vi "Dashboard Main.vi"() -> ()   [LabVIEW 2013]
uses:
  <vilib>/event_ctls.llb/eventvkey.ctl
  <vilib>/Rock Robotics/WPI/Dashboard/WPI_DashboardLogging Global.vi
  <vilib>/Utility/config.llb/Write Key (String).vi
  <vilib>/Utility/config.llb/Write Key (I32).vi
  <vilib>/Utility/config.llb/NI_LVConfig.lvlib
panel:
  out "Image Message":string="Timeout in Camera Communications"
  in  "Rec Mode":enum32{"Stop", "Record", "Playback"}(radio)
  in  "Dashboard Tab":T1(tab)
  out "right Encoder":dbl
  out "left Encoder":dbl
  out "Mode":string
  out "Timer":dbl
  in  "Camera Settings":T2={"Frame Rate"=30, "Compression"=30, "Size"=1} {"Frame Rate" scale=1.0..30.0; "Size" items=["640x480", "320x240", "160x120"]}
  out "MotorSliders R":cluster{"MotorSlide1":dbl, "MotorSlide2":dbl} {"MotorSlide2" scale=-1.0..1.0 scale format="%#_2e"; "MotorSlide1" scale=-1.0..1.0 scale format="%#_2e"}
  out "MotorChart R":cluster{"Numeric":dbl, "Numeric":dbl}(graph)
  out "MotorSliders L":T3 {"MotorSlide4 2" scale=0.0..14.0 scale format="%#_2e"; "MotorSlide2" scale=-1.0..1.0 scale format="%#_2e"; "MotorSlide1" scale=-1.0..1.0 scale format="%#_2e"}
  out "MotorChart L":T4(graph)
  out "JS1 Z":dbl(slide) scale=-1.0..1.0 scale format="%#_2e"
  out "Joystick 1":cluster{"X":dbl, "Y":dbl}[](graph)
  out "JS Buttons 1":T5
  out "JS2 Z":dbl(slide) scale=-1.0..1.0 scale format="%#_2e"
  out "Joystick 2":cluster{"X":dbl, "Y":dbl}[](graph)
  out "JS Buttons 2":T5
  out "Mode":T6(ring)=enum."Auto Disabled"
  out "Camera IP":string
  in  "DB Camera Config":bool
  out "fps":dbl format="%#.1g"
  out "Mbps":dbl format="%#.1g"
  out "Mbps 2":bool
  out "LED 1":bool
  out "Polt 2 Ind":dbl
  out "Plot 1 Ind":dbl
  out "Plot 0 Ind":dbl
  out "Waveform Chart":T7(graph)
  in  "Checkbox 2":bool
  in  "Checkbox 1":bool
  in  "Test Slider":dbl(slide) scale=0.0..100.0 scale format="%#_3g"
  in  "On/Off":bool caption="Solenoid"
  in  "Test Name":u16(ring) items=["Select the test to run...", "Example Test", "-------------------------------", "List of tests is built in robot code.", "Replace with your own automated tests."]
  in  "Test Tree":string(tree)
  in  "Motor":cluster{"Value":dbl, "Enable":bool} {"Value" scale=-1.0..1.0 scale format="%#_3g"}
  out "Progress":T8 {"Test Progress" scale=0.0..100.0}
  in  "Rev/Fwd":cluster{"Forward":bool, "Reverse":bool}
  in  "Test Ring":u16(ring) items=["Auto", "Fixed indoor", "Fixed outdoor 1", "Fixed outdoor 2", "Fixed fluorescent 1", "Fixed fluorescent 2", "Hold current"]
  in  "Listbox":i32(listbox)
  out "Tree":string(tree)
  out "Camera Image":T9(plugin-control)
  in  "Enable":bool
  # "Left"
  # "Front"
  # "Right"
  # "Battery"
  # "This tab is a great place for autonomous settings and validation.\nCustomize by placing controls and indicators here and name to\nmatch Dashboard Variables on robot."
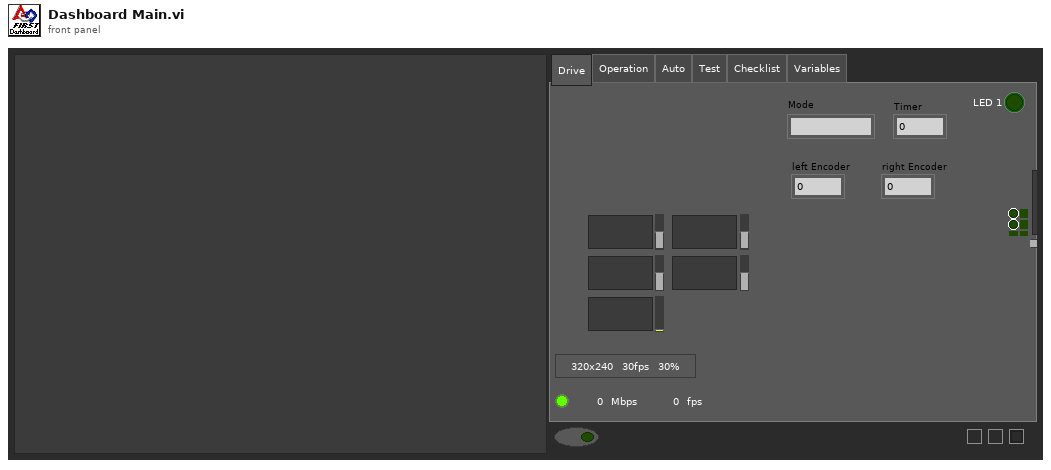
[diagram p1: front panel]
types:
  T1 = enum32{"Drive", "Operation", "Auto", "Test", "Checklist", "Variables"}
  T2 = cluster{"Frame Rate":i32, "Compression":i32, "Size":u16}
  T3 = cluster{"MotorSlide1":dbl, "MotorSlide2":dbl, "MotorSlide4 2":dbl}
  T4 = cluster{"Numeric":dbl, "Numeric":dbl, "Battery":sgl}
  T5 = cluster{bool, bool, bool, bool, bool, bool, bool, bool, bool, bool, bool, bool}
  T6 = enum8{"Tele-Op Disabled", "Tele-Op Enabled", "Auto Disabled", "Auto Enabled", "Test Disabled", "Test Enabled", ""}
  T7 = cluster{"Numeric":dbl, "Numeric":dbl, "Numeric":dbl}
  T8 = cluster{"Test Progress":u8, "Test Progress Text":string}
  T9 = typedef "IMAQ Image.ctl" = refnum<image>
  T10 = typedef "Image Type" = u32
  T11 = cluster{"Digital Inputs":bool[], "Digital Outputs":bool[]}
  T12 = cluster{"Competition mode":bool, "Robot Link":bool, "Autonomous":bool, "Enabled":bool, "E-Stop":bool, "Simulated":bool, "TestMode":bool, "Docked Window":bool}
  T13 = cluster{"Boolean":bool, "Boolean":bool, "Boolean":bool, "Boolean":bool, "Boolean":bool, "Boolean":bool, "Boolean":bool, "Boolean":bool, "Boolean":bool, "Boolean":bool, "Boolean":bool, "Boolean":bool}
  T14 = typedef "NI_LVConfig.lvlib/Config Data RefNum.ctl" = refnum<k1>
  T15 = typedef "eventvkey.ctl" = enum16{"ASCII", "Enter", "Return", "Shift", "Ctrl", "Alt", "Cmd", "Opt", "Caps", "NumLock", "Clear", "Break", "Up", "Down", "Left", "Right", "Insert", "Delete", "Home", "End", "PageUp", "PageDown", "Escape", "Help", "Pause", "ScrollLock", "F1", "F2", "F3", "F4", "F5", "F6", "F7", "F8", "F9", "F10", "F11", "F12", "F13", "F14", "F15", "F16", "F17", "F18", "F19", "F20", "F21", "F22", "F23", "F24", "Play", "VolumeUp", "VolumeDown", "Mute", "Two Byte Char"}
  T16 = cluster{"Image Size":bool, "Image Type":bool, "Pixel Value":bool, "ROI Information":bool, "Zoom Factor":bool}
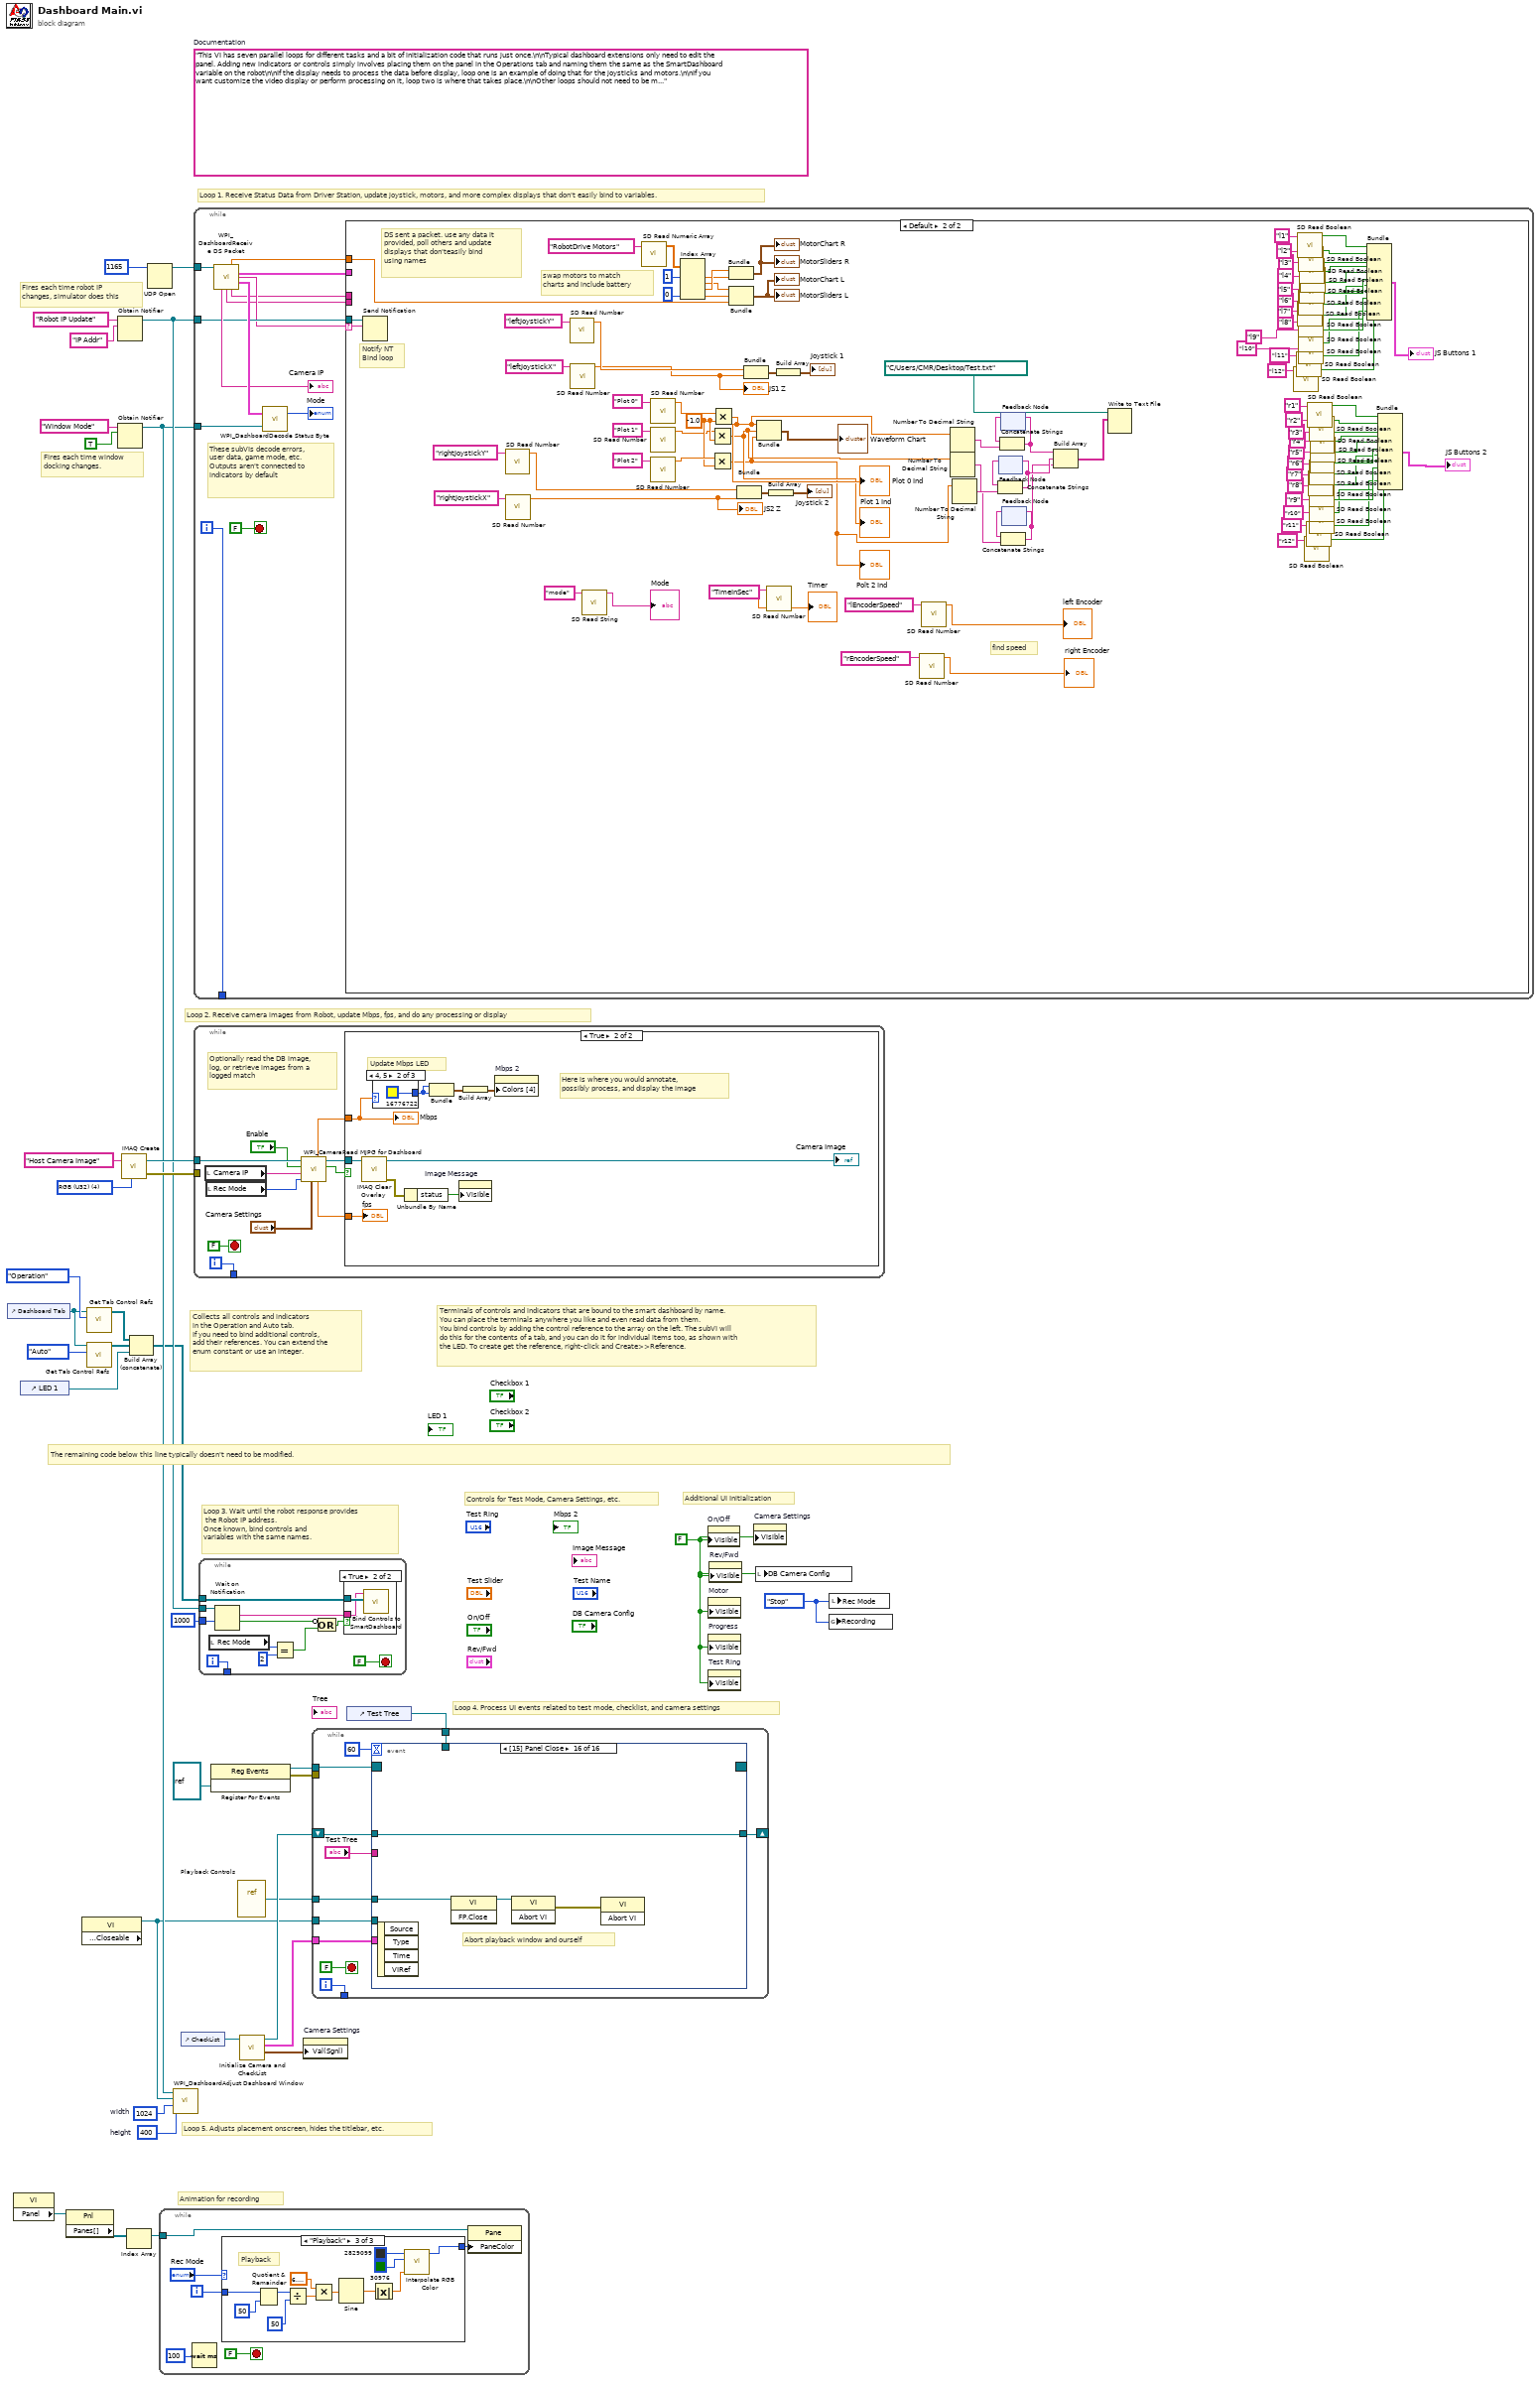
[diagram p0: block diagram]
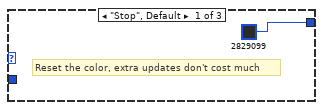
[diagram p2: hidden frame]
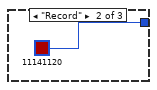
[diagram p3: hidden frame]
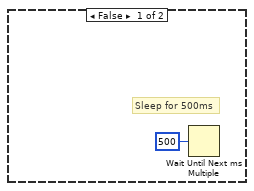
[diagram p5: hidden frame]
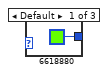
[diagram p6: hidden frame]
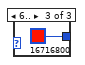
[diagram p7: hidden frame]
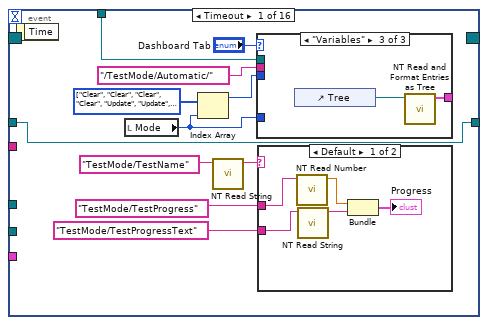
[diagram p8: hidden frame]
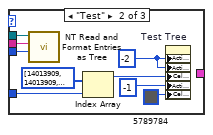
[diagram p10: hidden frame]
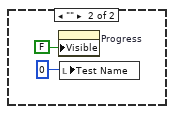
[diagram p11: hidden frame]
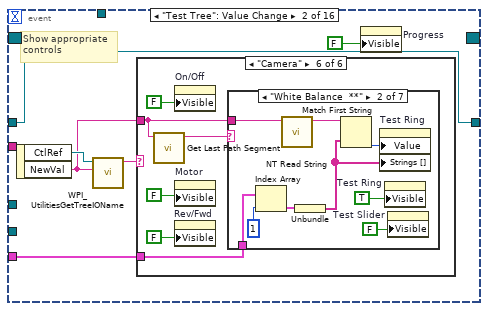
[diagram p12: hidden frame]
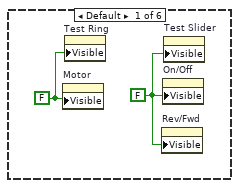
[diagram p13: hidden frame]
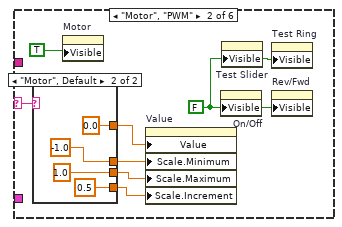
[diagram p14: hidden frame]
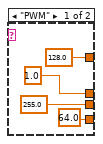
[diagram p15: hidden frame]
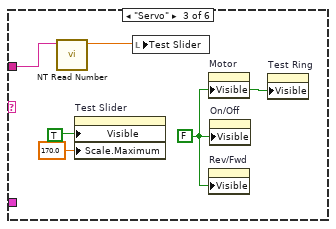
[diagram p16: hidden frame]
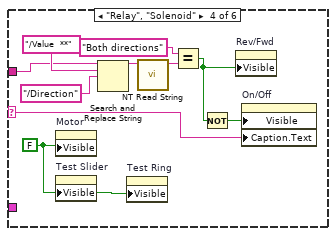
[diagram p17: hidden frame]
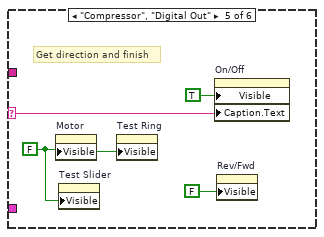
[diagram p18: hidden frame]
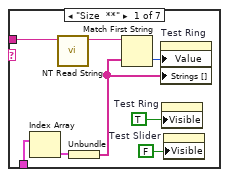
[diagram p19: hidden frame]
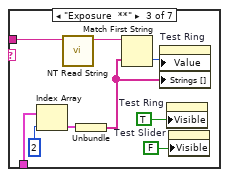
[diagram p20: hidden frame]
diagram:
  w8 = enum32{"Stop", "Record", "Playback"}."Stop" ("Rec Mode")
  w11 = 400  # height
  w12 = 1024  # width
  w25 = FALSE ("Visible")
  (unwired) "This VI has seven parallel loops for different tasks and a bit of initialization code that runs just once.\n\nTypical dashboard extensions only need to edit the panel. Adding new indicators or controls simply involves placing them on the panel in the Operations tab and naming them the same as the SmartDashboard variable on the robot\n\nIf the display needs to process the data before display, loop one is an example of doing that for the joysticks and motors.\n\nIf you want customize the video display or perform processing on it, loop two is where that takes place.\n\nOther loops should not need to be modified. They are pretty standard, and document the task they perform."  # Documentation
  w35 = T10 4 items=["Grayscale (U8)", "Grayscale (I16)", "Grayscale (SGL)", "Complex (CSG)", "RGB (U32)", "HSL (U32)", "RGB (U64)"] ("Image Type")
  # "Controls for Test Mode, Camera Settings, etc."
  # "Additional UI Initialization"
  # "Animation for recording"
  # "Fires each time robot IP\nchanges, simulator does this"
  # "Fires each time window\ndocking changes."
  # "Collects all controls and indicators\nin the Operation and Auto tab.\nIf you need to bind additional controls,\nadd their references. You can extend the\nenum constant or use an integer."
  # "The remaining code below this line typically doesn't need to be modified."
  # "Loop 4. Process UI events related to test mode, checklist, and camera settings"
  # "Terminals of controls and indicators that are bound to the smart dashboard by name.\nYou can place the terminals anywhere you like and even read data from them.\nYou bind controls by adding the control reference to the array on the left. The subVI will\ndo this for the contents of a tab, and you can do it for individual items too, as shown with\nthe LED. To create get the reference, right-click and Create>>Reference."
  # "Loop 3. Wait until the robot response provides\n the Robot IP address.\nOnce known, bind controls and\nvariables with the same names."
  # "Loop 5. Adjusts placement onscreen, hides the titlebar, etc."
  # "Loop 1. Receive Status Data from Driver Station, update joystick, motors, and more complex displays that don't easily bind to variables."
  # "Loop 2. Receive camera images from Robot, update Mbps, fps, and do any processing or display"
  n1 = control-ref of="Dashboard Tab"() -> (w6:refnum<vi>)
  n2 = property class="VI"() -> ("Panel"=w19:refnum<vi>)  [unwired: 2 in, 2 out]
  n3 = control-ref of="LED 1"() -> (w1:refnum<vi>)
  n4 = property class="Pnl"(reference=w19) -> ("Panes[]"=w20:refnum<vi>[])  [unwired: 1 in, 2 out]
  n5 = property class="VI" props=["Front Panel.Closeable"]() -> (reference out=w7:refnum<vi>)  [unwired: 2 in, 2 out]
  n6 = call <vilib>:"Get Tab Control Refs.vi"("Page Index"=T1."Operation" ("Dashboard Tab"), "TabControl in"=w6) -> ("ControlsOnPage"=w4:refnum<vi>[])  [unwired: 9 in]
  n7 = call <vilib>:"Get Tab Control Refs.vi"("Page Index"=T1."Auto" ("Dashboard Tab"), "TabControl in"=w6) -> ("ControlsOnPage"=w5:refnum<vi>[])  [unwired: 9 in]
  n8 = Obtain Notifier(name (unnamed)="Robot IP Update", notification data type="IP Addr" ("name (unnamed)")) -> (notifier out=w29:refnum<notifier>)  [unwired: 2 in, 2 out]
  n9 = Obtain Notifier(name (unnamed)="Window Mode", notification data type=TRUE) -> (notifier out=w10:refnum<notifier>)  [unwired: 2 in, 2 out]
  n10 = call "IMAQ Create"("Image Name"="Host Camera Image", "Image Type"=w35) -> ("New Image"=w33:T9, "error out"=w32:errorcluster)  [unwired: 2 in, 1 out]
  n11 = Index Array(array=w20) -> (element=w18:refnum<vi>)  [unwired: 1 in]
  n12 = Build Array (concatenate)(w4, w5, w1) -> (w3:refnum<vi>[])
  n13 = UDP Open(11:u16 1165 ("port")) -> (port=w36:refnum<k16>)  [unwired: 2 in, 4 out]
  n14 = while {
    tunnel: w18 -> [w39]
    i -> [w42]
    stop <- FALSE stop-if-true
    n15 = Wait (ms)(milliseconds to wait=u32 100) -> ()  [unwired: 1 out]
    n16 = case shown="\"Playback\"" "Rec Mode" {
      tunnel: w42 -> [_ _ w57]
      tunnel: [u32 2829099 ("Base Color") u32 11141120 ("Target Color") w46] -> w38
      frame "Stop", Default {
        # "Reset the color, extra updates don't cost much"
      }
      frame "Record" {
      }
      frame "Playback" {
        # "Playback"
        n17 = Quotient & Remainder(x=w57, y=u32 50 ("milliseconds to wait")) -> (x-y*floor(x/y)=w53:u32)  [unwired: 1 out]
        n18 = Divide(x=w53, y=u32 50 ("milliseconds to wait")) -> (x/y=w50:dbl)
        n19 = Multiply(x=6.283185307179586, y=w50) -> (x*y=w55:dbl)
        n20 = Sine(x=w55) -> (sin(x)=w54:dbl)
        n21 = Absolute Value(x=w54) -> (abs(x)=w47:dbl)
        n22 = call "Interpolate RGB Color.vi"("Proportion"=w47, "Target Color"=u32 30976, "Base Color"=u32 2829099) -> ("Result Color"=w46:u32)  [unwired: 8 in]
      }
    }
    n23 = property class="Pane"(reference=w39, "PaneColor"=w38) -> ()  [unwired: 1 in, 2 out]
  }
  n24 = call <vilib>:"WPI_DashboardAdjust Dashboard Window.vi"("height"=w11, "width"=w12, "reference in"=w7, "Notifier in"=w10) -> ()  [unwired: 8 in]
  n25 = control-ref of="CheckList"() -> (w9:refnum<vi>)
  n26 = while {
    tunnel: w33 -> [w66]
    tunnel: w32 -> [_]
    tunnel: [w67] -> _
    i -> [w67]
    stop <- FALSE stop-if-true
    # "Optionally read the DB image,\nlog, or retrieve images from a\nlogged match"
    n27 = local read "Camera IP"() -> (w59:string)
    n28 = local read "Rec Mode"() -> (w58:enum32{"Stop", "Record", "Playback"})
    n29 = call <vilib>:"WPI_CameraRead MJPG for Dashboard.vi"("Camera Settings"="Camera Settings", "Rec Mode"=w58, "Camera IP"=w59, "Enable"="Enable", "Refnum in"=w66) -> ("Active"=w63:bool, "Refnum out"=w65:T9, "FPS"=w62:dbl, "Bandwidth (Mbps)"=w61:dbl)  [unwired: 3 in]
    n30 = case shown="True" w63 {
      tunnel: w65 -> [_ w73]
      tunnel: w61 -> [_ w72]
      tunnel: w62 -> [_ w70]
      frame False {
        # "Sleep for 500ms"
        n31 = Wait Until Next ms Multiple(millisecond multiple=u32 500) -> ()  [unwired: 1 out]
      }
      frame True {
        # "Here is where you would annotate,\npossibly process, and display the image"
        # "Update Mbps LED"
        n32 = call "IMAQ Clear Overlay"("Image"=w73) -> ("error out"=w77:errorcluster, "Image Out"=→"Camera Image":T9)  [unwired: 2 in, 7 out]
        n33 = case shown="4, 5" w72 {
          tunnel: [u32 6618880 ("Color Box") u32 16776722 ("Color Box") u32 16716800 ("Color Box")] -> w74
          frame Default {
          }
          frame 4, 5 {
          }
          frame 6.. {
          }
        }
        n34 = Unbundle By Name(w77) -> ("status"=w78:bool)
        n35 = Bundle("Color Box"=w74, "Color Box"=w74) -> (w76:cluster{"Color Box":u32, "Color Box":u32})  [unwired: 1 out]
        n36 = property on="Image Message" class="Str"("Visible"=w78) -> ()  [unwired: 2 in, 2 out]
        n37 = Build Array(w76) -> (w75:cluster{"Color Box":u32, "Color Box":u32}[])
        n38 = property on="Mbps 2" class="Bool (strict)"("Colors [4]"=w75) -> ()  [unwired: 2 in, 2 out]
        "Mbps" <- w72
        "fps" <- w70
      }
    }
  }
  n39 = while {
    tunnel: w36 -> [w92]
    tunnel: w29 -> [w87]
    tunnel: w10 -> [w91]
    tunnel: [w88] -> _
    i -> [w88]
    stop <- FALSE stop-if-true
    # "These subVIs decode errors, user data, game mode, etc.\nOutputs aren't connected to indicators by default"
    n40 = call <vilib>:"WPI_DashboardReceive DS Packet.vi"("Recv Socket"=w92) -> ("Battery"=w82:sgl, "Driver Station"=w83:T11, "Robot IP Address"=w86:string, "Status"=w93:T12, "Camera IP Address"=→"Camera IP":string, "Low Priority User Data"=w85:string, "High Priority User Data"=w84:string)  [unwired: 1 in, 7 out]
    n41 = call <vilib>:"WPI_DashboardDecode Status Byte.vi"("Window Mode Notifier"=w91, "Status"=w93) -> ("Mode"=→"Mode":T6)  [unwired: 1 out]
    n42 = case shown="Default" w86 {
      selector: w86 -> [_ w193]
      tunnel: w87 -> [_ w194]
      tunnel: w85 -> [_ _]
      tunnel: w84 -> [_ _]
      tunnel: w83 -> [_ _]
      tunnel: w82 -> [_ w192]
      frame "0.0.0.0" {
        # "DS not sending packets, or no robot exists yet.\nDon't poll the variables"
      }
      frame Default {
        w111 = -1.0 ("y")
        # "find speed"
        # "Notify NT\nBind loop"
        # "DS sent a packet. use any data it\nprovided, poll others and update\ndisplays that don'teasily bind\nusing names"
        # "swap motors to match\ncharts and include battery"
        n43 = Send Notification(notification=w193, notifier=w194) -> ()  [unwired: 1 in, 2 out]
        n44 = call <vilib>:"SD Read Number.vi"("Name"="rightJoystickY") -> ("Numeric"=w114:dbl)  [unwired: 8 in, 2 out]
        n45 = call <vilib>:"SD Read Number.vi"("Name"="rightJoystickX") -> ("Numeric"=w178:dbl)  [unwired: 8 in, 2 out]
        "JS2 Z" <- w178
        n46 = call <vilib>:"SD Read Number.vi"("Name"="leftJoystickY") -> ("Numeric"=w177:dbl)  [unwired: 8 in, 2 out]
        n47 = call <vilib>:"SD Read Number.vi"("Name"="leftJoystickX") -> ("Numeric"=w176:dbl)  [unwired: 8 in, 2 out]
        "JS1 Z" <- w176
        n48 = call <vilib>:"SD Read String.vi"("Name"="mode") -> ("String"=→"Mode":string)  [unwired: 8 in, 2 out]
        n49 = call <vilib>:"SD Read Numeric Array.vi"("Name"="RobotDrive Motors") -> ("Numeric Array"=w191:dbl[])  [unwired: 8 in, 2 out]
        n50 = call <vilib>:"SD Read Number.vi"("Name"="Plot 0") -> ("Numeric"=w113:dbl)  [unwired: 8 in, 2 out]
        n51 = call <vilib>:"SD Read Number.vi"("Name"="Plot 1") -> ("Numeric"=w109:dbl)  [unwired: 8 in, 2 out]
        n52 = call <vilib>:"SD Read Number.vi"("Name"="Plot 2") -> ("Numeric"=w112:dbl)  [unwired: 8 in, 2 out]
        n53 = Index Array(array=w191, index #1=1, index #4=0) -> (element #1=w187:dbl, element #2=w186:dbl, element #3=w188:dbl, element #4=w183:dbl)  [unwired: 2 in]
        n54 = Multiply(x=w109, y=w111) -> (x*y=w106:dbl)
        "Plot 1 Ind" <- w106
        n55 = Multiply(x=w112, y=w111) -> (x*y=w105:dbl)
        "Polt 2 Ind" <- w105
        n56 = Multiply(x=w113, y=w111) -> (x*y=w107:dbl)
        "Plot 0 Ind" <- w107
        n57 = Bundle("Numeric"=w188, "Numeric"=w187) -> (→"MotorChart R" →"MotorSliders R":cluster{"Numeric":dbl, "Numeric":dbl})  [unwired: 1 in]
        n58 = Bundle("Numeric"=w186, "Numeric"=w183, "Battery"=w192) -> (→"MotorChart L" →"MotorSliders L":T4)  [unwired: 1 in]
        n59 = Bundle("Numeric"=w114, "Numeric"=w178) -> (w196:cluster{"Numeric":dbl, "Numeric":dbl})  [unwired: 1 in]
        n60 = Bundle("Numeric"=w177, "Numeric"=w176) -> (w198:cluster{"Numeric":dbl, "Numeric":dbl})  [unwired: 1 in]
        n61 = Bundle(w107, w106, w105) -> (→"Waveform Chart":cluster{dbl, dbl, dbl})  [unwired: 1 in]
        n62 = call <vilib>:"SD Read Number.vi"("Name"="TimeInSec") -> ("Numeric"=→"Timer":dbl)  [unwired: 8 in, 2 out]
        n63 = Build Array(w196) -> (→"Joystick 2":cluster{"Numeric":dbl, "Numeric":dbl}[])
        n64 = Build Array(w198) -> (→"Joystick 1":cluster{"Numeric":dbl, "Numeric":dbl}[])
        n65 = call <vilib>:"SD Read Number.vi"("Name"="rEncoderSpeed") -> ("Numeric"=→"right Encoder":dbl)  [unwired: 8 in, 2 out]
        n66 = call <vilib>:"SD Read Number.vi"("Name"="lEncoderSpeed") -> ("Numeric"=→"left Encoder":dbl)  [unwired: 8 in, 2 out]
        n67 = Number To Decimal String(number=w107) -> (decimal integer string=w103:string)  [unwired: 1 in]
        n68 = Number To Decimal String(number=w106) -> (decimal integer string=w100:string)  [unwired: 1 in]
        n69 = Number To Decimal String(number=w105) -> (decimal integer string=w97:string)  [unwired: 1 in]
        n70 = feedback #1() -> (w101:string)  [unwired: 1 in]
        n71 = Concatenate Strings(w101, w100) -> (w99:string)
        n72 = feedback-in #1(w99) -> ()
        n73 = feedback #2() -> (w104:string)  [unwired: 1 in]
        n74 = Concatenate Strings(w104, w103) -> (w102:string)
        n75 = feedback-in #2(w102) -> ()
        n76 = feedback #3() -> (w98:string)  [unwired: 1 in]
        n77 = Concatenate Strings(w98, w97) -> (w96:string)
        n78 = feedback-in #3(w96) -> ()
        n79 = Build Array(w102, w99, w96) -> (w95:string[])
        n80 = Write to Text File(file (use dialog)=path "C:/Users/CMR/Desktop/Test.txt", text=w95) -> ()  [unwired: 2 in, 3 out]
        n81 = call <vilib>:"SD Read Boolean.vi"("Name"="l12") -> ("Boolean"=w152:bool)  [unwired: 8 in, 2 out]
        n82 = call <vilib>:"SD Read Boolean.vi"("Name"="l11") -> ("Boolean"=w153:bool)  [unwired: 8 in, 2 out]
        n83 = call <vilib>:"SD Read Boolean.vi"("Name"="l1") -> ("Boolean"=w163:bool)  [unwired: 8 in, 2 out]
        n84 = call <vilib>:"SD Read Boolean.vi"("Name"="l7") -> ("Boolean"=w157:bool)  [unwired: 8 in, 2 out]
        n85 = call <vilib>:"SD Read Boolean.vi"("Name"="l2") -> ("Boolean"=w162:bool)  [unwired: 8 in, 2 out]
        n86 = call <vilib>:"SD Read Boolean.vi"("Name"="l6") -> ("Boolean"=w158:bool)  [unwired: 8 in, 2 out]
        n87 = call <vilib>:"SD Read Boolean.vi"("Name"="l8") -> ("Boolean"=w156:bool)  [unwired: 8 in, 2 out]
        n88 = call <vilib>:"SD Read Boolean.vi"("Name"="l9") -> ("Boolean"=w155:bool)  [unwired: 8 in, 2 out]
        n89 = call <vilib>:"SD Read Boolean.vi"("Name"="l10") -> ("Boolean"=w154:bool)  [unwired: 8 in, 2 out]
        n90 = call <vilib>:"SD Read Boolean.vi"("Name"="l3") -> ("Boolean"=w161:bool)  [unwired: 8 in, 2 out]
        n91 = call <vilib>:"SD Read Boolean.vi"("Name"="l5") -> ("Boolean"=w159:bool)  [unwired: 8 in, 2 out]
        n92 = call <vilib>:"SD Read Boolean.vi"("Name"="l4") -> ("Boolean"=w160:bool)  [unwired: 8 in, 2 out]
        n93 = call <vilib>:"SD Read Boolean.vi"("Name"="r12") -> ("Boolean"=w164:bool)  [unwired: 8 in, 2 out]
        n94 = call <vilib>:"SD Read Boolean.vi"("Name"="r11") -> ("Boolean"=w165:bool)  [unwired: 8 in, 2 out]
        n95 = call <vilib>:"SD Read Boolean.vi"("Name"="r1") -> ("Boolean"=w175:bool)  [unwired: 8 in, 2 out]
        n96 = call <vilib>:"SD Read Boolean.vi"("Name"="r7") -> ("Boolean"=w169:bool)  [unwired: 8 in, 2 out]
        n97 = call <vilib>:"SD Read Boolean.vi"("Name"="r2") -> ("Boolean"=w174:bool)  [unwired: 8 in, 2 out]
        n98 = call <vilib>:"SD Read Boolean.vi"("Name"="r6") -> ("Boolean"=w170:bool)  [unwired: 8 in, 2 out]
        n99 = call <vilib>:"SD Read Boolean.vi"("Name"="r8") -> ("Boolean"=w168:bool)  [unwired: 8 in, 2 out]
        n100 = call <vilib>:"SD Read Boolean.vi"("Name"="r9") -> ("Boolean"=w167:bool)  [unwired: 8 in, 2 out]
        n101 = call <vilib>:"SD Read Boolean.vi"("Name"="r10") -> ("Boolean"=w166:bool)  [unwired: 8 in, 2 out]
        n102 = call <vilib>:"SD Read Boolean.vi"("Name"="r3") -> ("Boolean"=w173:bool)  [unwired: 8 in, 2 out]
        n103 = call <vilib>:"SD Read Boolean.vi"("Name"="r5") -> ("Boolean"=w171:bool)  [unwired: 8 in, 2 out]
        n104 = call <vilib>:"SD Read Boolean.vi"("Name"="r4") -> ("Boolean"=w172:bool)  [unwired: 8 in, 2 out]
        n105 = Bundle("Boolean"=w163, "Boolean"=w162, "Boolean"=w161, "Boolean"=w160, "Boolean"=w159, "Boolean"=w158, "Boolean"=w157, "Boolean"=w156, "Boolean"=w155, "Boolean"=w154, "Boolean"=w153, "Boolean"=w152) -> (→"JS Buttons 1":T13)  [unwired: 1 in]
        n106 = Bundle("Boolean"=w175, "Boolean"=w174, "Boolean"=w173, "Boolean"=w172, "Boolean"=w171, "Boolean"=w170, "Boolean"=w169, "Boolean"=w168, "Boolean"=w167, "Boolean"=w166, "Boolean"=w165, "Boolean"=w164) -> (→"JS Buttons 2":T13)  [unwired: 1 in]
      }
    }
  }
  n107 = while {
    tunnel: w3 -> [w210]
    tunnel: w29 -> [w208]
    tunnel: [w206] -> _
    tunnel: u32 1000 ("milliseconds to wait") -> [w205]
    i -> [w206]
    stop <- FALSE stop-if-true
    n108 = local read "Rec Mode"() -> (w201:enum32{"Stop", "Record", "Playback"})
    n109 = Wait on Notification(notifier=w208, timeout in ms (-1)=w205) -> (notification=w207:string, timed out?=w203:bool)  [unwired: 2 in, 2 out]
    n110 = Equal?(x=w201, y=u16 2 ("Rec Mode")) -> (x = y?=w202:bool)
    n111 = Compound Arithmetic op=OR(invert w203, w202) -> (w204:bool)
    n112 = case shown="True" w204 {
      tunnel: w210 -> [_ w212]
      tunnel: w207 -> [_ w211]
      frame False {
      }
      frame True {
        n113 = call <vilib>:"Bind Controls to SmartDashboard.vi"("Bound Control Refs"=w212, "Server IP Address"=w211) -> ()  [unwired: 10 in]
      }
    }
  }
  n114 = register-events(refnum<vi> refnum) -> (reference out=w16:refnum<event-registration>, error out=w15:errorcluster)  [unwired: 2 in]
  n115 = vi-ref "Playback Controls.vi"() -> (w17:refnum<vi>)
  n116 = call "Initialize Camera and CheckList.vi"("ListBox in"=w9) -> ("Cluster"=w23:cluster{"value":i32, "value":i32, "index":i32}, "Array"=w24:cluster{string[]}[], "File Refnum"=w22:T14)  [unwired: 8 in]
  n117 = property on="Camera Settings" class="Clust (strict)"("Val(Sgnl)"=w23) -> ()  [unwired: 2 in, 2 out]
  n118 = control-ref of="Test Tree"() -> (w21:refnum<vi>)
  n119 = while {
    tunnel: w24 -> [w220]
    shift-right: [w219] -> _
    shift-left: w22 -> [w218]
    tunnel: [w217] -> _
    tunnel: w21 -> [w216]
    tunnel: w17 -> [w215]
    tunnel: w16 -> [w214]
    tunnel: w15 -> [_]
    tunnel: w7 -> [w213]
    i -> [w217]
    stop <- FALSE stop-if-true
    n120 = event shown="[15] Panel Close" {
      selector: w214 -> [_ _ _ _ _ _ _ _ _ _ _ _ _ _ _ _]
      dyn-events: [_ _ _ _ _ _ _ _ _ _ _ _ _ w458 _ _] -> _
      timeout: u32 60 ("milliseconds to wait") -> [_ _ _ _ _ _ _ _ _ _ _ _ _ _ _ _]
      tunnel: w216 -> [w230 _ _ _ _ _ _ _ _ _ _ _ _ _ _ _]
      tunnel: "Test Tree" -> [_ _ _ _ _ _ _ _ w427 w435 w437 w441 w449 _ _ _]
      tunnel: w220 -> [_ w254 _ _ _ _ w391 w421 _ _ _ _ _ _ _ _]
      tunnel: [w224 w253 w352 w357 w365 w377 w390 w414 w426 w433 w436 w440 w448 w460 w474 w475] -> w219
      tunnel: w218 -> [w224 w253 w352 w357 w365 w377 w389 w414 w426 w433 w436 w440 w448 w460 w474 w475]
      tunnel: w215 -> [_ _ _ _ _ _ _ _ _ _ _ _ _ w461 _ w478]
      tunnel: w213 -> [_ _ _ _ _ _ _ _ _ _ _ _ _ w456 _ _]
      event Timeout {
        w229 = enum16{"Update", "Clear"}[] [enum."Clear", enum."Clear", enum."Clear", enum."Clear", enum."Update", enum."Update", enum."Clear"] items=["Update", "Clear"]
        n121 = event-data() -> ()  [unwired: 1 in, 1 out]
        n122 = local read "Mode"() -> (w227:T6)
        n123 = Index Array(array=w229, index=w227) -> (element=w228:enum16{"Update", "Clear"})
        n124 = call <vilib>:"NT Read String.vi"("Name"="TestMode/TestName") -> ("String"=w233:string)  [unwired: 9 in, 1 out]
        n125 = case shown="\"Variables\"" "Dashboard Tab" {
          tunnel: w230 -> [_ w243 _]
          tunnel: "/TestMode/Automatic/" ("Name Pattern") -> [_ w242 _]
          tunnel: w228 -> [_ w241 _]
          tunnel: w227 -> [_ w239 _]
          tunnel: [_ _ w245] -> _
          frame "Operation", Default {
          }
          frame "Test" {
            w238 = -2 ("Active Item:Row Number")
            n126 = call <vilib>:"NT Read and Format Entries as Tree.vi"("Operation"=w241, "Name Pattern"=w242, "Tree Refnum"=w243) -> ()  [unwired: 7 in, 2 out]
            n127 = Index Array(array=u32[] [14013909, 14013909, 14013909, 14013909, 14013909, 16777215, 14013909], index=w239) -> (element=w237:u32)
            n128 = property on="Test Tree" class="Tree (strict)"("Active Item Row Number"=w238, "ActiveColNum"=w238, "CellBG"=w237, "Active Item Row Number"=-1 ("Active Item:Row Number"), "CellBG"=u32 5789784 ("Color Box")) -> ()  [unwired: 2 in, 2 out]
          }
          frame "Variables" {
            n129 = control-ref of="Tree"() -> (w244:refnum<vi>)
            n130 = call <vilib>:"NT Read and Format Entries as Tree.vi"("Tree Refnum"=w244) -> ("Formatted Strings"=w245:cluster{"Name":string, "Value":string}[])  [unwired: 9 in, 1 out]
          }
        }
        n131 = case shown="Default" w233 {
          tunnel: "TestMode/TestProgress" ("Name") -> [w247 _]
          tunnel: "TestMode/TestProgressText" ("Name") -> [w246 _]
          frame Default {
            n132 = call <vilib>:"NT Read Number.vi"("Name"=w247) -> ("Numeric"=w248:dbl)  [unwired: 9 in, 1 out]
            n133 = call <vilib>:"NT Read String.vi"("Name"=w246) -> ("String"=w249:string)  [unwired: 9 in, 1 out]
            n134 = Bundle("Numeric"=w248, "String"=w249) -> (→"Progress":cluster{"Numeric":dbl, "String":string})  [unwired: 1 in]
          }
          frame "" {
            n135 = property on="Progress" class="Clust (strict)"("Visible"=FALSE) -> ()  [unwired: 2 in, 2 out]
            n136 = local write "Test Name"(u16 0) -> ()
          }
        }
      }
      event "Test Tree": Value Change {
        # "Show appropriate\ncontrols"
        n137 = event-data() -> ("CtlRef"=w257:refnum<vi>, "NewVal"=w255:string)  [unwired: 1 in]
        n138 = call <vilib>:"WPI_UtilitiesGetTreeIOName.vi"("NewVal"=w255, "TreeControl in"=w257) -> ("I/O Name"=w258:string)  [unwired: 9 in]
        n139 = case shown="\"Camera\"" w258 {
          selector: w258 -> [_ w265 _ w283 w292 _]
          tunnel: w255 -> [_ _ w280 w282 _ w299]
          tunnel: w254 -> [_ _ _ _ _ w298]
          frame Default {
            w260 = FALSE ("Visible")
            w259 = FALSE ("Visible")
            n140 = property on="Motor" class="Clust (strict)"("Visible"=w259) -> ()  [unwired: 2 in, 2 out]
            n141 = property on="Test Ring" class="Ring (strict)"("Visible"=w259) -> ()  [unwired: 2 in, 2 out]
            n142 = property on="Rev/Fwd" class="Clust (strict)"("Visible"=w260) -> ()  [unwired: 2 in, 2 out]
            n143 = property on="On/Off" class="Bool (strict)"("Visible"=w260) -> ()  [unwired: 2 in, 2 out]
            n144 = property on="Test Slider" class="Slide (strict)"("Visible"=w260) -> ()  [unwired: 2 in, 2 out]
          }
          frame "Motor", "PWM" {
            w266 = FALSE ("Visible")
            n145 = case shown="\"Motor\", Default" w265 {
              tunnel: [1.0 ("Value") -1.0 ("Value")] -> w264
              tunnel: [255.0 ("Value") 1.0 ("Value")] -> w263
              tunnel: [128.0 ("Value") 0.0 ("Value")] -> w262
              tunnel: [64.0 ("Value") 0.5 ("Value")] -> w261
              frame "PWM" {
              }
              frame "Motor", Default {
              }
            }
            n146 = property on="Motor" class="Clust (strict)"("Visible"=TRUE) -> ()  [unwired: 2 in, 2 out]
            n147 = property on="Value" class="Slide (strict)"("Value"=w262, "Scale.Minimum"=w264, "Scale.Maximum"=w263, "Scale.Increment"=w261) -> ()  [unwired: 2 in, 2 out]
            n148 = property on="On/Off" class="Bool (strict)"("Visible"=w266) -> ()  [unwired: 2 in, 2 out]
            n149 = property on="Test Slider" class="Slide (strict)"("Visible"=w266) -> ()  [unwired: 2 in, 2 out]
            n150 = property on="Test Ring" class="Ring (strict)"("Visible"=w266) -> ()  [unwired: 2 in, 2 out]
            n151 = property on="Rev/Fwd" class="Clust (strict)"("Visible"=w266) -> ()  [unwired: 2 in, 2 out]
          }
          frame "Servo" {
            w278 = FALSE ("Visible")
            n152 = call <vilib>:"NT Read Number.vi"("Name"=w280) -> ("Numeric"=w279:dbl)  [unwired: 9 in, 1 out]
            n153 = property on="Test Slider" class="Slide (strict)"("Visible"=TRUE, "Scale.Maximum"=170.0 ("Scale.Range:Maximum")) -> ()  [unwired: 2 in, 2 out]
            n154 = local write "Test Slider"(w279) -> ()
            n155 = property on="Motor" class="Clust (strict)"("Visible"=w278) -> ()  [unwired: 2 in, 2 out]
            n156 = property on="Rev/Fwd" class="Clust (strict)"("Visible"=w278) -> ()  [unwired: 2 in, 2 out]
            n157 = property on="On/Off" class="Bool (strict)"("Visible"=w278) -> ()  [unwired: 2 in, 2 out]
            n158 = property on="Test Ring" class="Ring (strict)"("Visible"=w278) -> ()  [unwired: 2 in, 2 out]
          }
          frame "Relay", "Solenoid" {
            w281 = FALSE ("Visible")
            n159 = property on="Motor" class="Clust (strict)"("Visible"=w281) -> ()  [unwired: 2 in, 2 out]
            n160 = property on="Test Slider" class="Slide (strict)"("Visible"=w281) -> ()  [unwired: 2 in, 2 out]
            n161 = Search and Replace String(input string=w282, search string="/Value  **", replace string="/Direction") -> (result string=w288:string)  [unwired: 5 in, 3 out]
            n162 = property on="Test Ring" class="Ring (strict)"("Visible"=w281) -> ()  [unwired: 2 in, 2 out]
            n163 = call <vilib>:"NT Read String.vi"("Name"=w288) -> ("String"=w286:string)  [unwired: 9 in, 1 out]
            n164 = Equal?(x="Both directions", y=w286) -> (x = y?=w284:bool)
            n165 = Not(x=w284) -> (.not. x?=w285:bool)
            n166 = property on="Rev/Fwd" class="Clust (strict)"("Visible"=w284) -> ()  [unwired: 2 in, 2 out]
            n167 = property on="On/Off" class="Bool (strict)"("Visible"=w285, "Caption.Text"=w283) -> ()  [unwired: 2 in, 2 out]
          }
          frame "Compressor", "Digital Out" {
            w291 = FALSE ("Visible")
            # "Get direction and finish"
            n168 = property on="Motor" class="Clust (strict)"("Visible"=w291) -> ()  [unwired: 2 in, 2 out]
            n169 = property on="Test Slider" class="Slide (strict)"("Visible"=w291) -> ()  [unwired: 2 in, 2 out]
            n170 = property on="Test Ring" class="Ring (strict)"("Visible"=w291) -> ()  [unwired: 2 in, 2 out]
            n171 = property on="On/Off" class="Bool (strict)"("Visible"=TRUE, "Caption.Text"=w292) -> ()  [unwired: 2 in, 2 out]
            n172 = property on="Rev/Fwd" class="Clust (strict)"("Visible"=FALSE) -> ()  [unwired: 2 in, 2 out]
          }
          frame "Camera" {
            n173 = call <vilib>:"Get Last Path Segment.vi"("String in"=w299) -> ("String out"=w300:string)  [unwired: 10 in]
            n174 = property on="On/Off" class="Bool (strict)"("Visible"=FALSE) -> ()  [unwired: 2 in, 2 out]
            n175 = property on="Motor" class="Clust (strict)"("Visible"=FALSE) -> ()  [unwired: 2 in, 2 out]
            n176 = property on="Rev/Fwd" class="Clust (strict)"("Visible"=FALSE) -> ()  [unwired: 2 in, 2 out]
            n177 = case shown="\"White Balance  **\"" w300 {
              tunnel: w299 -> [w306 w315 w324 w333 w342 _ w348]
              tunnel: w298 -> [w304 w312 w321 w330 w339 _ _]
              frame "Size  **" {
                n178 = Index Array(array=w304) -> (element=w303:cluster{string[]})  [unwired: 1 in]
                n179 = call <vilib>:"NT Read String.vi"("Name"=w306) -> ("String"=w305:string)  [unwired: 9 in, 1 out]
                n180 = Unbundle(w303) -> (w301:string[])
                n181 = Match First String(2:w301, 3:w305) -> (0:w302:i32)  [unwired: 1 out]
                n182 = property on="Test Ring" class="Ring (strict)"("Value"=w302, "Strings []"=w301) -> ()  [unwired: 2 in, 2 out]
                n183 = property on="Test Ring" class="Ring (strict)"("Visible"=TRUE) -> ()  [unwired: 2 in, 2 out]
                n184 = property on="Test Slider" class="Slide (strict)"("Visible"=FALSE) -> ()  [unwired: 2 in, 2 out]
              }
              frame "White Balance  **" {
                n185 = Index Array(array=w312, index=1) -> (element=w313:cluster{string[]})
                n186 = call <vilib>:"NT Read String.vi"("Name"=w315) -> ("String"=w314:string)  [unwired: 9 in, 1 out]
                n187 = Unbundle(w313) -> (w310:string[])
                n188 = Match First String(2:w310, 3:w314) -> (0:w309:i32)  [unwired: 1 out]
                n189 = property on="Test Ring" class="Ring (strict)"("Value"=w309, "Strings []"=w310) -> ()  [unwired: 2 in, 2 out]
                n190 = property on="Test Ring" class="Ring (strict)"("Visible"=TRUE) -> ()  [unwired: 2 in, 2 out]
                n191 = property on="Test Slider" class="Slide (strict)"("Visible"=FALSE) -> ()  [unwired: 2 in, 2 out]
              }
              frame "Exposure  **" {
                n192 = Index Array(array=w321, index=2) -> (element=w322:cluster{string[]})
                n193 = call <vilib>:"NT Read String.vi"("Name"=w324) -> ("String"=w323:string)  [unwired: 9 in, 1 out]
                n194 = Unbundle(w322) -> (w318:string[])
                n195 = Match First String(2:w318, 3:w323) -> (0:w319:i32)  [unwired: 1 out]
                n196 = property on="Test Ring" class="Ring (strict)"("Value"=w319, "Strings []"=w318) -> ()  [unwired: 2 in, 2 out]
                n197 = property on="Test Ring" class="Ring (strict)"("Visible"=TRUE) -> ()  [unwired: 2 in, 2 out]
                n198 = property on="Test Slider" class="Slide (strict)"("Visible"=FALSE) -> ()  [unwired: 2 in, 2 out]
              }
              frame "Exposure Priority  **" {
                n199 = Index Array(array=w330, index=3) -> (element=w331:cluster{string[]})
                n200 = call <vilib>:"NT Read String.vi"("Name"=w333) -> ("String"=w332:string)  [unwired: 9 in, 1 out]
                n201 = Unbundle(w331) -> (w327:string[])
                n202 = Match First String(2:w327, 3:w332) -> (0:w328:i32)  [unwired: 1 out]
                n203 = property on="Test Ring" class="Ring (strict)"("Value"=w328, "Strings []"=w327) -> ()  [unwired: 2 in, 2 out]
                n204 = property on="Test Ring" class="Ring (strict)"("Visible"=TRUE) -> ()  [unwired: 2 in, 2 out]
                n205 = property on="Test Slider" class="Slide (strict)"("Visible"=FALSE) -> ()  [unwired: 2 in, 2 out]
              }
              frame "Color Enable  **" {
                n206 = Index Array(array=w339, index=4) -> (element=w340:cluster{string[]})
                n207 = call <vilib>:"NT Read String.vi"("Name"=w342) -> ("String"=w341:string)  [unwired: 9 in, 1 out]
                n208 = Unbundle(w340) -> (w336:string[])
                n209 = Match First String(2:w336, 3:w341) -> (0:w337:i32)  [unwired: 1 out]
                n210 = property on="Test Ring" class="Ring (strict)"("Value"=w337, "Strings []"=w336) -> ()  [unwired: 2 in, 2 out]
                n211 = property on="Test Ring" class="Ring (strict)"("Visible"=TRUE) -> ()  [unwired: 2 in, 2 out]
                n212 = property on="Test Slider" class="Slide (strict)"("Visible"=FALSE) -> ()  [unwired: 2 in, 2 out]
              }
              frame Default {
                n213 = property on="Test Ring" class="Ring (strict)"("Visible"=FALSE) -> ()  [unwired: 2 in, 2 out]
                n214 = property on="Test Slider" class="Slide (strict)"("Visible"=FALSE) -> ()  [unwired: 2 in, 2 out]
              }
              frame "Brightness  **", "Color Level  **", "Compression  **", "FPS  **", "Sharpness  **" {
                n215 = call <vilib>:"NT Read Number.vi"("Name"=w348) -> ("Numeric"=w347:dbl)  [unwired: 9 in, 1 out]
                n216 = local write "Test Slider"(w347) -> ()
                n217 = property on="Test Slider" class="Slide (strict)"("Visible"=TRUE, "Scale.Maximum"=100.0 ("Scale.Range:Maximum")) -> ()  [unwired: 2 in, 2 out]
                n218 = property on="Test Ring" class="Ring (strict)"("Visible"=FALSE) -> ()  [unwired: 2 in, 2 out]
              }
            }
          }
        }
        n219 = property on="Progress" class="Clust (strict)"("Visible"=FALSE) -> ()  [unwired: 2 in, 2 out]
      }
      event "Test Name": Mouse Enter {
        # "Populate the ring with the list of tests"
        n220 = event-data() -> ()  [unwired: 1 in, 1 out]
        n221 = call <vilib>:"NT Read String Array.vi"("Name"="TestMode/TestList") -> ("String Array"=w356:string[])  [unwired: 9 in, 1 out]
        n222 = Build Array (concatenate)("Select the test to run...", w356) -> (w355:string[])
        n223 = property on="Test Name" class="Ring (strict)"("Strings []"=w355) -> ()  [unwired: 2 in, 2 out]
      }
      event "Test Name": Value Change {
        w358 = FALSE ("Visible")
        # "Tell the robot the test name to run"
        n224 = event-data() -> ("NewVal"=w362:u16)  [unwired: 1 in]
        n225 = property on="Test Name" class="Ring (strict)"() -> ("Strings []"=w363:string[])  [unwired: 2 in, 2 out]
        n226 = local write "Progress"(T8 {"Test Progress"=0, "Test Progress Text"=""} ("Progress")) -> ()
        n227 = Index Array(array=w363, index=w362) -> (element=w361:string)
        n228 = call <vilib>:"NT Write String.vi"("String"=w361, "Name"="TestMode/TestName") -> ()  [unwired: 9 in, 1 out]
        n229 = property on="Progress" class="Clust (strict)"("Visible"=TRUE) -> ()  [unwired: 2 in, 2 out]
        n230 = property on="Motor" class="Clust (strict)"("Visible"=w358) -> ()  [unwired: 2 in, 2 out]
        n231 = property on="Test Slider" class="Slide (strict)"("Visible"=w358) -> ()  [unwired: 2 in, 2 out]
        n232 = property on="On/Off" class="Bool (strict)"("Visible"=w358) -> ()  [unwired: 2 in, 2 out]
        n233 = property on="Rev/Fwd" class="Clust (strict)"("Visible"=w358) -> ()  [unwired: 2 in, 2 out]
        n234 = property on="Test Ring" class="Ring (strict)"("Visible"=w358) -> ()  [unwired: 2 in, 2 out]
      }
      event "Listbox": Double Click {
        n235 = event-data() -> ("PlatMods.Shift"=w366:bool, "Row"=w368:i32)  [unwired: 1 in]
        n236 = case shown="True" w366 {
          tunnel: w368 -> [w372 _]
          tunnel: 1 -> [w371 _]
          frame False {
            n237 = property on="Listbox" class="LstBox (strict)"() -> ("Item Symbols"=w370:i32[])  [unwired: 2 in, 2 out]
            n238 = Replace Array Subset(array=w370, new element=w371, index=w372) -> (w369:i32[])
            n239 = property on="Listbox" class="LstBox (strict)"("Item Symbols"=w369) -> ()  [unwired: 2 in, 2 out]
          }
          frame True {
            w373 = 0 ("Top Row")
            n240 = property on="Listbox" class="LstBox (strict)"() -> ("Number of Rows"=w375:u32)  [unwired: 2 in, 2 out]
            n241 = Initialize Array(0, w375) -> (w374:i32[])
            n242 = property on="Listbox" class="LstBox (strict)"("Top Row"=w373, "Value"=w373, "Item Symbols"=w374) -> ()  [unwired: 2 in, 2 out]
          }
        }
      }
      event "Listbox": Key Down {
        n243 = event-data() -> ("VKey"=w379:T15)  [unwired: 1 in]
        n244 = case shown="\"Left\", \"Right\"" w379 {
          selector: w379 -> [w384 _]
          tunnel: eventvkey."Left" ("VKey") -> [w382 _]
          frame "Left", "Right" {
            n245 = Equal?(x=w382, y=w384) -> (x = y?=w383:bool)
            n246 = Select(t=0, s=w383, f=1) -> (s? t:f=w385:i32)
            n247 = property on="Listbox" class="LstBox (strict)"() -> ("Item Symbols"=w388:i32[])  [unwired: 2 in, 2 out]
            n248 = Replace Array Subset(array=w388, new element=w385, index="Listbox") -> (w387:i32[])
            n249 = property on="Listbox" class="LstBox (strict)"("Item Symbols"=w387) -> ()  [unwired: 2 in, 2 out]
          }
          frame Default {
          }
        }
      }
      event "DB Camera Config": Value Change {
        n250 = event-data() -> ("NewVal"=w392:bool)  [unwired: 1 in]
        n251 = case shown="False" w392 {
          tunnel: w391 -> [w401 _]
          tunnel: [w394 w412] -> w390
          tunnel: w389 -> [w393 w412]
          frame False {
            w408 = "Camera"
            w411 = FALSE ("Visible")
            n252 = local read "Camera Settings"() -> (w400:T2)
            n253 = Index Array(array=w401) -> (element=w404:cluster{string[]})  [unwired: 1 in]
            n254 = Unbundle(w400) -> ("Frame Rate"=w399:i32, "Compression"=w398:i32, "Size"=w402:u16)
            n255 = Unbundle(w404) -> (w403:string[])
            n256 = Index Array(array=w403, index=w402) -> (element=w397:string)
            n257 = call-poly <vilib>:"Write Key.vi"("section"=w408, "value"=w397, "key"="Size", "refnum"=w393) -> ("refnum out"=w410:T14)  [unwired: 2 in, 5 out]
            n258 = call-poly <vilib>:"Write Key.vi"("section"=w408, "value"=w399, "key"="FrameRate", "refnum"=w410) -> ("refnum out"=w409:T14)  [unwired: 1 in, 6 out]
            n259 = property on="Camera Settings" class="Clust (strict)"("Visible"=w411) -> ()  [unwired: 2 in, 2 out]
            n260 = local write "DB Camera Config"(w411) -> ()
            n261 = call-poly <vilib>:"Write Key.vi"("section"=w408, "value"=w398, "key"="Compression", "refnum"=w409) -> ("refnum out"=w395:T14)  [unwired: 1 in, 6 out]
            n262 = call <vilib>:"Close Config Data.vi"("refnum"=w395) -> ("file path"=w396:path)  [unwired: 2 in, 8 out]
            n263 = call <vilib>:"Open Config Data.vi"("configuration file path"=w396) -> ("refnum"=w394:T14)  [unwired: 8 in, 2 out]
          }
          frame True {
            n264 = property on="Camera Settings" class="Clust (strict)"("Visible"=TRUE) -> ()  [unwired: 2 in, 2 out]
          }
        }
      }
      event "Camera Settings": Value Change {
        n265 = event-data() -> ("NewVal"=w425:T2)  [unwired: 1 in]
        n266 = Index Array(array=w421) -> (element=w420:cluster{string[]})  [unwired: 1 in]
        n267 = Unbundle(w425) -> ("Frame Rate"=w416:i32, "Compression"=w415:i32, "Size"=w418:u16)
        n268 = Unbundle(w420) -> (w419:string[])
        n269 = Index Array(array=w419, index=w418) -> (element=w417:string)
        n270 = Format Into String(format string="%s   %dfps   %d%%", w417, w416, w415) -> (resulting string=w422:string)  [unwired: 2 in, 1 out]
        n271 = Build Array(w422) -> (w423:string[])
        n272 = property on="DB Camera Config" class="Bool (strict)"("Strings [4]"=w423) -> ()  [unwired: 2 in, 2 out]
      }
      event "Motor.Enable": Value Change {
        n273 = event-data() -> ("NewVal"=w431:bool)  [unwired: 1 in]
        n274 = Unbundle("Motor") -> ("Value"=w430:dbl)  [unwired: 1 out]
        n275 = Select(t=w430, s=w431, f=0.0) -> (s? t:f=w428:dbl)
        n276 = call <vilib>:"NT Write Number.vi"("Numeric"=w428, "Name"=w427) -> ()  [unwired: 9 in, 1 out]
      }
      event "Test Slider": Value Change {
        n277 = event-data() -> ("NewVal"=w434:dbl)  [unwired: 1 in]
        n278 = call <vilib>:"NT Write Number.vi"("Numeric"=w434, "Name"=w435) -> ()  [unwired: 9 in, 1 out]
      }
      event "On/Off": Value Change {
        n279 = event-data() -> ("NewVal"=w439:bool)  [unwired: 1 in]
        n280 = Boolean To (0,1)(Boolean=w439) -> (0, 1=w438:i16)
        n281 = call <vilib>:"NT Write Number.vi"("Numeric"=w438, "Name"=w437) -> ()  [unwired: 9 in, 1 out]
      }
      event "Rev/Fwd": Value Change {
        n282 = event-data() -> ("NewVal.Forward"=w447:bool, "NewVal.Reverse"=w446:bool)  [unwired: 1 in]
        n283 = Boolean To (0,1)(Boolean=w447) -> (0, 1=w443:i16)
        n284 = Boolean To (0,1)(Boolean=w446) -> (0, 1=w445:i16)
        n285 = Negate(x=w445) -> (-x=w444:i16)
        n286 = Add(x=w443, y=w444) -> (x+y=w442:i16)
        n287 = call <vilib>:"NT Write Number.vi"("Numeric"=w442, "Name"=w441) -> ()  [unwired: 9 in, 1 out]
      }
      event "Test Ring": Value Change {
        n288 = event-data() -> ("NewVal"=w451:u16)  [unwired: 1 in]
        n289 = property on="Test Ring" class="Ring (strict)"() -> ("Strings []"=w452:string[])  [unwired: 2 in, 2 out]
        n290 = Index Array(array=w452, index=w451) -> (element=w450:string)
        n291 = call <vilib>:"NT Write String.vi"("String"=w450, "Name"=w449) -> ()  [unwired: 9 in, 1 out]
      }
      event "Rec Mode": Value Change {
        # "Update globals for recording mode and path to read log from.\nClear when logging and let NetworkTables set path for vision to\nuse."
        n292 = event-data() -> ("NewVal"=w462:enum32{"Stop", "Record", "Playback"})  [unwired: 1 in]
        n293 = global write "WPI_DashboardLogging Global.vi" "Logging Filename"(path "") -> ()
        n294 = case shown="\"Stop\", \"Record\"" w462 {
          tunnel: w461 -> [_ w464 w472]
          tunnel: [_ _ w471] -> w458
          tunnel: [_ _ w470] -> _
          tunnel: w456 -> [_ _ w468]
          tunnel: cluster{i32, i32} {-250, 170} -> [_ _ w467]
          tunnel: [_ _ T16 {"Image Size"=TRUE, "Image Type"=TRUE, "Pixel Value"=TRUE, "ROI Information"=TRUE, "Zoom Factor"=FALSE} ("Image Information Shown:All Elements")] -> w454
          tunnel: [_ _ TRUE ("Zoom Factor")] -> w453
          frame Default {
          }
          frame "Stop", "Record" {
            # "Place Window too"
            n295 = invoke class="VI" method="FP.Close"(reference=w464) -> (reference out=w463:refnum<vi>)  [unwired: 2 in, 2 out]
            n296 = invoke class="VI" method="Abort VI"(reference=w463) -> ()  [unwired: 2 in, 3 out]
          }
          frame "Playback" {
            n297 = call "Open Playback Panel.vi"("Offset"=w467, "DB VI Ref"=w468, "Playback in"=w472) -> ("Playback out"=w469:refnum<vi>)  [unwired: 8 in]
            n298 = register-events(w469) -> (reference out=w471:refnum<event-registration>, error out=w470:errorcluster)  [unwired: 2 in]
          }
        }
        n299 = global write "WPI_DashboardLogging Global.vi" "Recording"(w462) -> ()
        n300 = property on="Camera Image" class="ImageControl"("Image Information Shown"=w454, "Image Information Visible"=w453) -> ()  [unwired: 2 in, 2 out]
        n301 = call <vilib>:"WPI_DashboardNT Log FieldName Cache.vi"("Operation"=enum16{"Lookup/Add", "Index", "Clear"}."Clear") -> ()  [unwired: 8 in, 3 out]
      }
      event Panel Close {
        w473 = enum32{"Stop", "Record", "Playback"}."Stop" ("Rec Mode")
        n302 = event-data() -> ()  [unwired: 1 in, 4 out]
        n303 = local write "Rec Mode"(w473) -> ()
        n304 = global write "WPI_DashboardLogging Global.vi" "Recording"(w473) -> ()
      }
      event Panel Close {
        # "Abort playback window and ourself"
        n305 = event-data() -> ()  [unwired: 1 in, 4 out]
        n306 = invoke class="VI" method="FP.Close"(reference=w478) -> (reference out=w477:refnum<vi>)  [unwired: 2 in, 2 out]
        n307 = invoke class="VI" method="Abort VI"(reference=w477) -> (error out=w476:errorcluster)  [unwired: 2 in, 2 out]
        n308 = invoke class="VI" method="Abort VI"(error in=w476) -> ()  [unwired: 2 in, 3 out]
      }
    }
  }
  n309 = property on="On/Off" class="Bool (strict)"("Visible"=w25) -> ()  [unwired: 2 in, 2 out]
  n310 = property on="Motor" class="Clust (strict)"("Visible"=w25) -> ()  [unwired: 2 in, 2 out]
  n311 = property on="Progress" class="Clust (strict)"("Visible"=w25) -> ()  [unwired: 2 in, 2 out]
  n312 = property on="Test Ring" class="Ring (strict)"("Visible"=w25) -> ()  [unwired: 2 in, 2 out]
  n313 = property on="Rev/Fwd" class="Clust (strict)"("Visible"=w25) -> ()  [unwired: 2 in, 2 out]
  n314 = property on="Camera Settings" class="Clust (strict)"("Visible"=w25) -> ()  [unwired: 2 in, 2 out]
  n315 = local write "DB Camera Config"(w25) -> ()
  n316 = global write "WPI_DashboardLogging Global.vi" "Recording"(w8) -> ()
  n317 = local write "Rec Mode"(w8) -> ()
